vi "up2uw.vi"(2 "error in (no error)":errorcluster, 3 "up":dbl) -> (0 "error out":errorcluster, 1 "uw":dbl)   [LabVIEW 2021]
panel:
  out "b":dbl=-64.3266
  out "a":dbl=0.0696
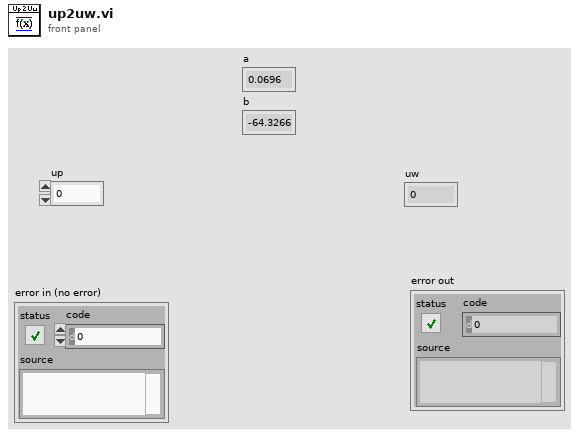
[diagram p1: front panel]
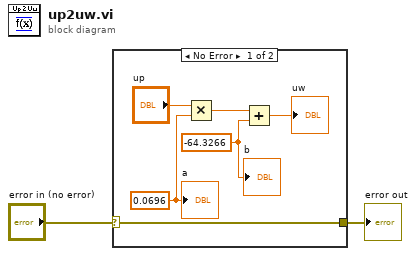
[diagram p0: block diagram]
diagram:
  n1 = case shown="No Error" "error in (no error)" {
    selector: "error in (no error)" -> [w8 w9]
    tunnel: [w8 w9] -> w2
    frame No Error {
      w4 = -64.3266 ("y")
      w6 = 0.0696 ("y")
      n2 = Multiply(x="up", y=w6) -> (x*y=w5:dbl)
      n3 = Add(x=w5, y=w4) -> (x+y=→"uw":dbl)
      "a" <- w6
      "b" <- w4
    }
    frame Error {
    }
  }
  "error out" <- w2
